vi "Show MiniGUI.vi"(8 "error in (no error)":errorcluster, 10 "MiniGUI Index":i32, 11 "LabGUI in":refnum<class "LabGUI.lvclass">) -> (0 "error out":errorcluster, 3 "LabGUI out":refnum<class "LabGUI.lvclass">)   [LabVIEW 2019, in "LabGUI.lvlib" / "LabGUI.lvclass"]
uses:
  LabGUI.lvclass
  LabGUI.lvclass/LabGUI.ctl
  MiniGUI/MiniGUI Messages/Get IP Msg/Read RT Dataset Msg.lvclass/Read RT Dataset Msg.ctl
  <vilib>/ActorFramework/Message Enqueuer/Message Enqueuer.lvclass/Message Enqueuer.ctl
  <vilib>/ActorFramework/Message Enqueuer/Enqueue.vi
  MiniGUI/MiniGUI Messages/Get IP Msg/Read RT Dataset Msg.lvclass
  C:/Program Files (x86)/National Instruments/LabVIEW 2019/vi.lib/ActorFramework/Message/Message.lvclass
  <vilib>/ActorFramework/Message Priority Queue/Priority Enqueue.vi
  <vilib>/MGI/Panel Manager/Panel Actor/Panel Actor Messages/Show Panel Msg/Show Panel Msg.lvclass
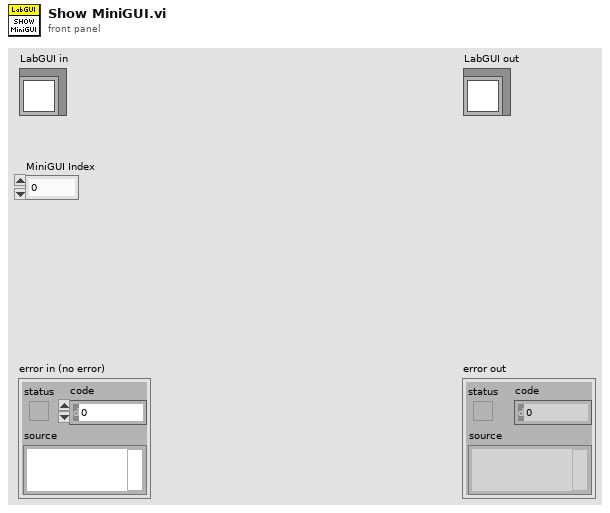
[diagram p1: front panel]
types:
  T1 = map{string, refnum<class "Message Enqueuer.lvclass">}
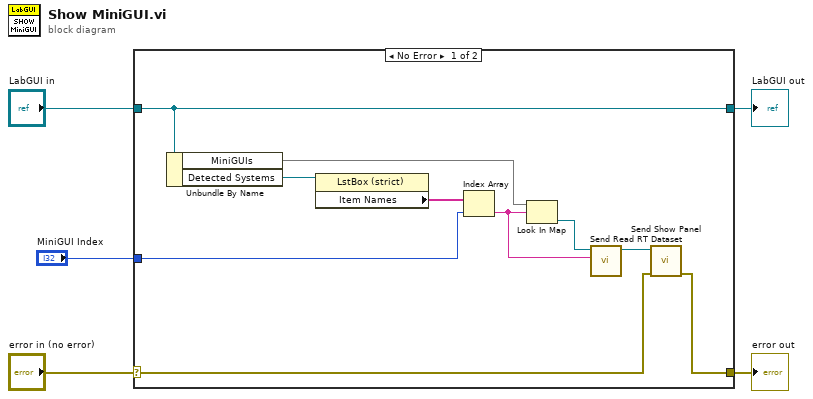
[diagram p0: block diagram]
diagram:
  n1 = case shown="No Error" "error in (no error)" {
    selector: "error in (no error)" -> [w10 w17]
    tunnel: [w9 w17] -> w4
    tunnel: [w15 w16] -> w2
    tunnel: "LabGUI in" -> [w15 w16]
    tunnel: "MiniGUI Index" -> [w11 _]
    frame No Error {
      n2 = Unbundle By Name(w15) -> ("MiniGUIs"=w14:T1, "Detected Systems"=w13:refnum<vi>)
      n3 = property class="LstBox (strict)"(reference=w13) -> ("Item Names"=w12:string[])  [unwired: 1 in, 2 out]
      n4 = Index Array(array=w12, index=w11) -> (element=w6:string)
      n5 = Look In Map(map=w14, key=w6) -> (value=w8:refnum<class "Message Enqueuer.lvclass">)  [unwired: 1 in, 1 out]
      n6 = call "Send Read RT Dataset.vi"("IP Address"=w6, "Message Enqueuer"=w8) -> ("Message Enqueuer out"=w7:refnum<class "Message Enqueuer.lvclass">)  [unwired: 8 in, 1 out]
      n7 = call <vilib>:"Send Show Panel.vi"("Error In"=w10, "Message Enqueuer in"=w7) -> ("Error Out"=w9:errorcluster)  [unwired: 8 in, 1 out]
    }
    frame Error {
    }
  }
  "error out" <- w4
  "LabGUI out" <- w2
